vi "读取生成cover.vi"(8 "error in (no error)":errorcluster caption="错误输入（无错误）", 11 "EPUB输入":refnum<class "EPUB.lvclass">) -> (0 "error out":errorcluster caption="错误输出", 2 "cover":string, 3 "EPUB输出":refnum<class "EPUB.lvclass">)   [LabVIEW 2016, in "EPUB.lvclass"]
uses:
  EPUB.lvclass
  EPUB.lvclass/EPUB.ctl
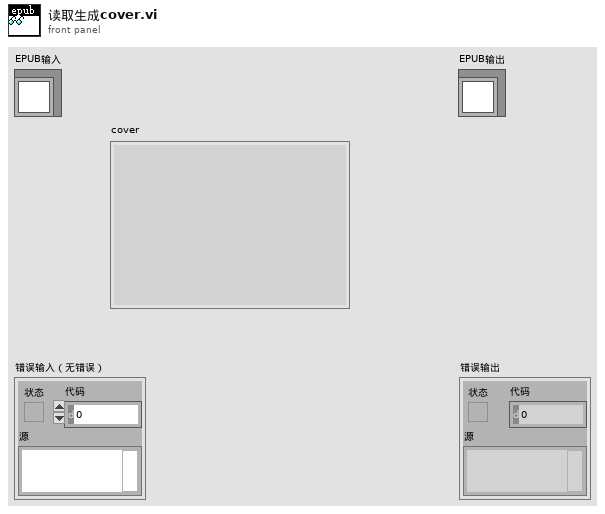
[diagram p1: front panel]
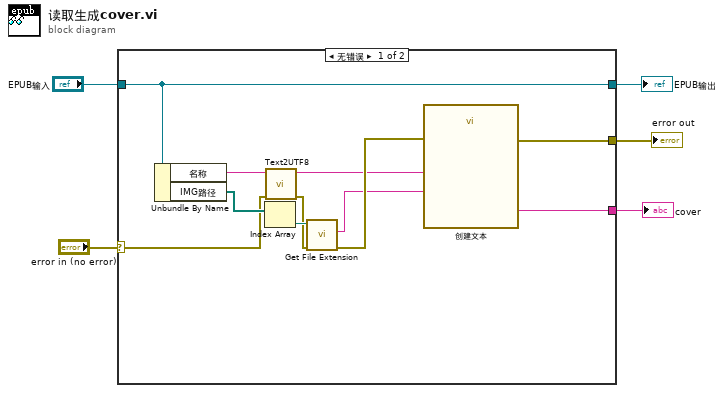
[diagram p0: block diagram]
diagram:
  n1 = case shown="无错误" "error in (no error)" {
    selector: "error in (no error)" -> [w6 w17]
    tunnel: [w15 w17] -> w4
    tunnel: [w16 w18] -> w2
    tunnel: "EPUB输入" -> [w16 w18]
    tunnel: [w12 _] -> w1
    frame No Error {
      n2 = Unbundle By Name(w16) -> ("名称"=w8:string, "IMG路径"=w13:path[])
      n3 = Index Array(array=w13) -> (element=w11:path)  [unwired: 1 in]
      n4 = call <vilib>:"Text2UTF8.vi"("Error in"=w6, "text"=w8) -> ("Error out"=w7:errorcluster, "utf-8 text"=w9:string)  [unwired: 8 in]
      n5 = call <vilib>:"Get File Extension.vi"("error in (no error)"=w7, "file"=w11) -> ("error out"=w14:errorcluster, "lowercase file extension"=w10:string)  [unwired: 5 in, 3 out]
      n6 = call "创建文本"("title"=w9, "extname"=w10, "error in (no error)"=w14) -> ("Result"=w12:string, "error out"=w15:errorcluster)  [unwired: 11 in]
    }
    frame Error {
    }
  }
  "error out" <- w4
  "EPUB输出" <- w2
  "cover" <- w1
